vi "Start Sync.vi"(8 "error in (no error)":errorcluster, 11 "gRPC service in":refnum<class "OOBgRPCService.lvclass">) -> (0 "error out":errorcluster, 3 "gRPC service out":refnum<class "OOBgRPCService.lvclass">)   [LabVIEW 2025, in "OOB gRPC Server.lvlib" / "OOBgRPCService.lvclass"]
uses:
  OOBgRPCService.lvclass
  OOBgRPCService.lvclass/OOBgRPCService.ctl
  OOB Data Transfer/OOB Data Transfer.lvlib
  RPC Messages/hwval_GenericResponse.ctl
  OOB gRPC Server.lvlib
  RPC Messages/hwval_StatusResponse.ctl
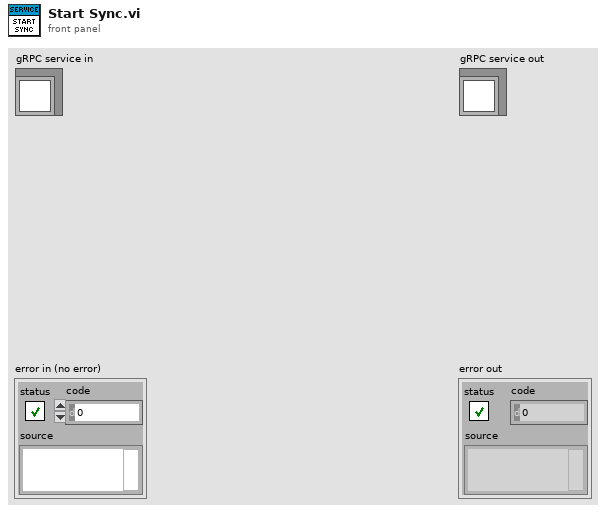
[diagram p1: front panel]
types:
  T1 = typedef "OOB gRPC Server.lvlib/hwval_GenericResponse.ctl" = cluster{"Payload":u8[]}
  T2 = typedef "OOB gRPC Server.lvlib/hwval_StatusResponse.ctl" = cluster{"Status":bool, "Code":i32, "Message":string}
  T3 = typedef "OOB gRPC Server.lvlib/OOBgRPCService.lvclass/Server Internal UEs.ctl" = cluster{"OOBgRPCService Generic Internal UE":refnum<user-event>, "OOBgRPCService PauseResume Internal UE":refnum<user-event>, "OOBgRPCService Export Internal UE":refnum<user-event>}
  T4 = typedef "OOB gRPC Server.lvlib/OOBgRPCService.lvclass/Server gRPC UEs.ctl" = cluster{"OOBgRPCService Generic gRPC UE":refnum<user-event>, "OOBgRPCService PauseResume gRPC UE":refnum<user-event>, "OOBgRPCService Export gRPC UE":refnum<user-event>}
  T5 = typedef "grpc-lvsupport-release.lvlib/grpcId.ctl" = u64
  T6 = typedef "OOB gRPC Server.lvlib/hwval_GenericRequest.ctl" = cluster{"Command":string, "Payload":u8[]}
  T7 = typedef "OOB Data Transfer.lvlib/OOB to Logic Data.ctl" = cluster{"PauseResume":bool, "Export":string}
  T8 = typedef "OOB gRPC Server.lvlib/hwval_BoolRequest.ctl" = cluster{"BooleanData":bool}
  T9 = typedef "OOB gRPC Server.lvlib/hwval_ExportRequest.ctl" = cluster{"FileType":string}
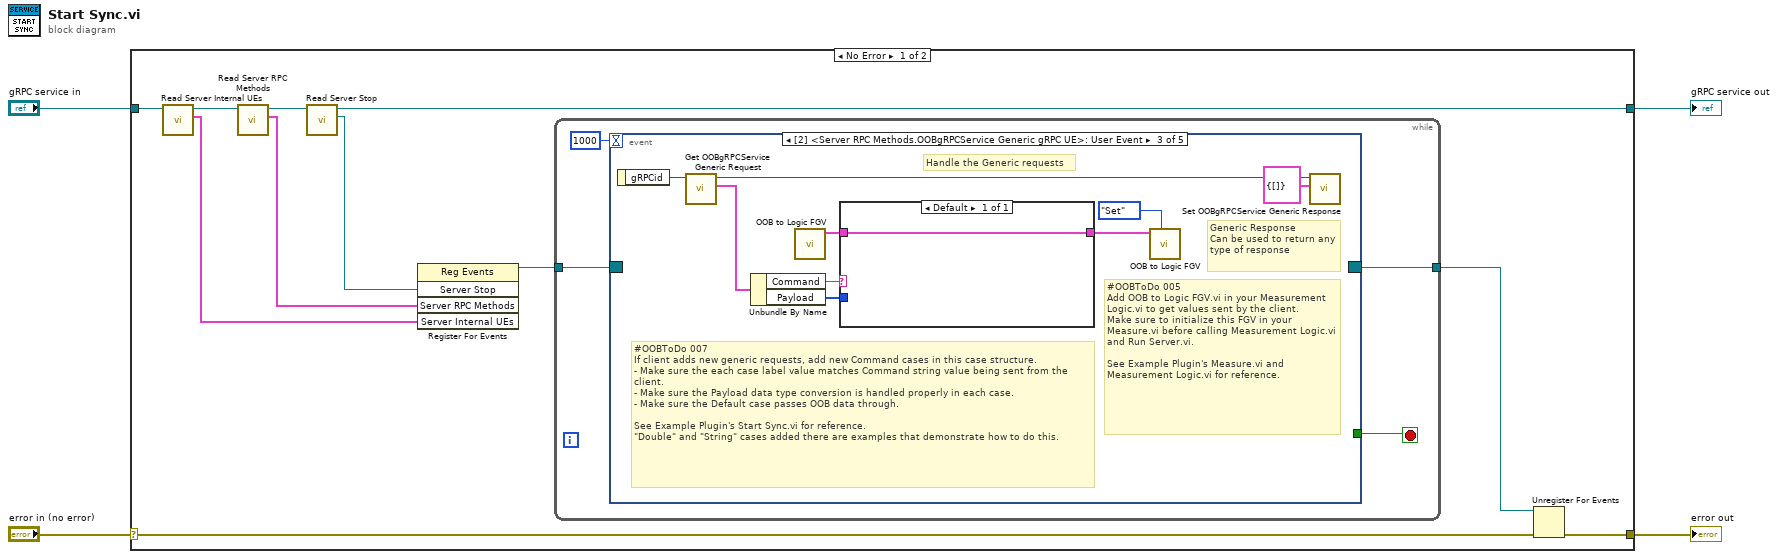
[diagram p0: block diagram]
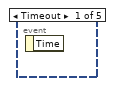
[diagram p2: hidden frame]
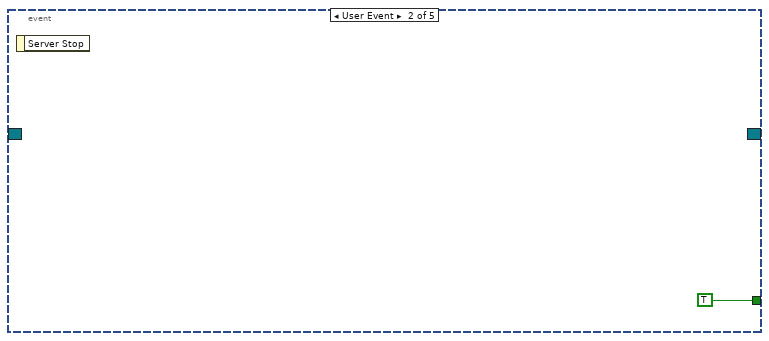
[diagram p3: hidden frame]
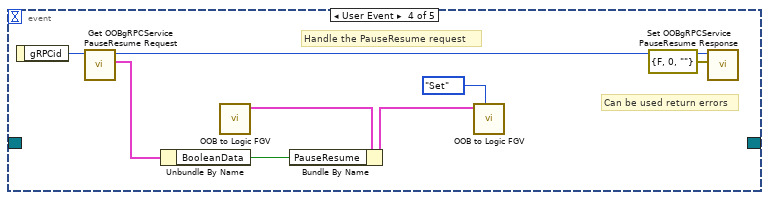
[diagram p4: hidden frame]
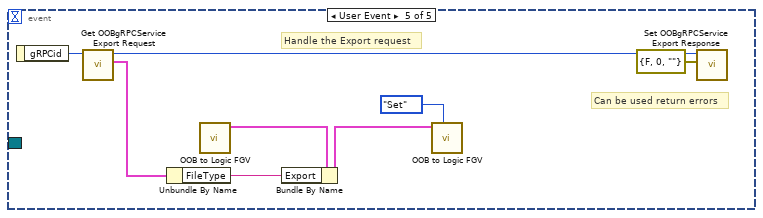
[diagram p5: hidden frame]
diagram:
  n1 = case shown="No Error" "error in (no error)" {
    selector: "error in (no error)" -> [w9 w48]
    tunnel: [w8 w48] -> w3
    tunnel: [w6 w47] -> w1
    tunnel: "gRPC service in" -> [w15 w47]
    frame No Error {
      n2 = call "Read Server Internal UEs.vi"("gRPC service in"=w15) -> ("Server Internal UEs"=w13:T3, "gRPC service out"=w14:refnum<class "OOBgRPCService.lvclass">)  [unwired: 8 in, 1 out]
      n3 = call "Read Server RPC Methods.vi"("gRPC service in"=w14) -> ("Server RPC Methods"=w7:T4, "gRPC service out"=w12:refnum<class "OOBgRPCService.lvclass">)  [unwired: 8 in, 1 out]
      n4 = call-dynamic "Read Server Stop.vi"("gRPC service in"=w12) -> ("Server Stop"=w5:refnum<user-event>, "gRPC service out"=w6:refnum<class "OOBgRPCService.lvclass">)  [unwired: 8 in, 1 out]
      n5 = register-events(w5, w7, w13) -> (reference out=w11:refnum<event-registration>)  [unwired: 2 in, 1 out]
      n6 = while {
        tunnel: w11 -> [w19]
        tunnel: [w17] -> w10
        stop <- w18 stop-if-true
        n7 = event "RPC Methods Event Structure" shown="[2] <Server RPC Methods.OOBgRPCService Generic gRPC UE>: User Event" {
          selector: w19 -> [_ _ _ _ _]
          dyn-events: [_ _ _ _ _] -> w17
          timeout: 1000 -> [_ _ _ _ _]
          tunnel: [_ TRUE _ _ _] -> w18
          event Timeout {
            n8 = event-data() -> ()  [unwired: 1 in, 1 out]
          }
          event User Event {
            n9 = event-data() -> ()  [unwired: 1 in, 1 out]
          }
          event User Event {
            # "#OOBToDo 007 \nIf client adds new generic requests, add new Command cases in this case structure. \n- Make sure the each case label value matches Command string value being sent from the client.\n- Make sure the Payload data type conversion is handled properly in each case.\n- Make sure the Default case passes OOB data through.\n\nSee Example Plugin's Start Sync.vi for reference. \n\"Double\" and \"String\" cases added there are examples that demonstrate how to do this."
            # "Handle the Generic requests"
            # "Generic Response\nCan be used to return any type of response"
            # "#OOBToDo 005 \nAdd OOB to Logic FGV.vi in your Measurement Logic.vi to get values sent by the client.\nMake sure to initialize this FGV in your Measure.vi before calling Measurement Logic.vi and Run Server.vi.\n\nSee Example Plugin's Measure.vi and Measurement Logic.vi for reference."
            n10 = event-data() -> ("gRPCid"=w29:T5)  [unwired: 1 in]
            n11 = call "Get OOBgRPCService Generic Request.vi"("gRPCid"=w29) -> ("Message Data"=w27:T6, "gRPCid out"=w28:T5)  [unwired: 8 in, 1 out]
            n12 = Unbundle By Name(w27) -> ("Command"=w22:string, "Payload"=w21:u8[])
            n13 = call "OOB to Logic FGV.vi"() -> ("OOB to Logic Data out"=w24:T7)  [unwired: 10 in, 1 out]
            n14 = case shown="Default" w22 {
              tunnel: w24 -> [w30]
              tunnel: [w30] -> w23
              tunnel: w21 -> [_]
              frame Default {
              }
            }
            n15 = call "OOB to Logic FGV.vi"("Op (Get)"=enum16{"Get", "Set"}."Set", "OOB to Logic Data in"=w23) -> ()  [unwired: 8 in, 2 out]
            n16 = call "Set OOBgRPCService Generic Response.vi"("Message Data"=T1 {"Payload"=[]}, "gRPCid in"=w28) -> ()  [unwired: 9 in, 1 out]
          }
          event User Event {
            # "Handle the PauseResume request"
            # "Can be used return errors"
            n17 = event-data() -> ("gRPCid"=w32:T5)  [unwired: 1 in]
            n18 = call "Get OOBgRPCService PauseResume Request.vi"("gRPCid"=w32) -> ("Message Data"=w34:T8, "gRPCid out"=w35:T5)  [unwired: 8 in, 1 out]
            n19 = Unbundle By Name(w34) -> ("BooleanData"=w33:bool)
            n20 = call "OOB to Logic FGV.vi"() -> ("OOB to Logic Data out"=w37:T7)  [unwired: 10 in, 1 out]
            n21 = Bundle By Name(cluster=w37, "PauseResume"=w33) -> (w36:T7)
            n22 = call "OOB to Logic FGV.vi"("Op (Get)"=enum16{"Get", "Set"}."Set", "OOB to Logic Data in"=w36) -> ()  [unwired: 8 in, 2 out]
            n23 = call "Set OOBgRPCService PauseResume Response.vi"("Message Data"=T2 {"Status"=FALSE, "Code"=0, "Message"=""}, "gRPCid in"=w35) -> ()  [unwired: 9 in, 1 out]
          }
          event User Event {
            # "Handle the Export request"
            # "Can be used return errors"
            n24 = event-data() -> ("gRPCid"=w40:T5)  [unwired: 1 in]
            n25 = call "Get OOBgRPCService Export Request.vi"("gRPCid"=w40) -> ("Message Data"=w42:T9, "gRPCid out"=w46:T5)  [unwired: 8 in, 1 out]
            n26 = Unbundle By Name(w42) -> ("FileType"=w41:string)
            n27 = call "OOB to Logic FGV.vi"() -> ("OOB to Logic Data out"=w44:T7)  [unwired: 10 in, 1 out]
            n28 = Bundle By Name(cluster=w44, "Export"=w41) -> (w43:T7)
            n29 = call "OOB to Logic FGV.vi"("Op (Get)"=enum16{"Get", "Set"}."Set", "OOB to Logic Data in"=w43) -> ()  [unwired: 8 in, 2 out]
            n30 = call "Set OOBgRPCService Export Response.vi"("Message Data"=T2 {"Status"=FALSE, "Code"=0, "Message"=""}, "gRPCid in"=w46) -> ()  [unwired: 9 in, 1 out]
          }
        }
      }
      n31 = Unregister For Events(event registration refnum=w10, error in=w9) -> (error out=w8:errorcluster)
    }
    frame Error {
    }
  }
  "error out" <- w3
  "gRPC service out" <- w1
